vi "CH_LM Globals Debug-Status.vi"() -> ()   [LabVIEW 2017, in "CH_LM App.lvlib"]
uses:
  CH_LM App.lvlib
panel:
  in  "Load Reference":refnum<vi>
  out "Log Counter":i32
  out "GUI Counter":i32
  out "Calculate Counter":i32
  out "Fetch Counter":i32
  out "Callback Counter":i32
  out "Bytes per Element - Trend":i32
  out "Bytes per Element - Log":i32
  out "Bytes per Element - Stream":i32
  in  "My Reference":refnum<vi>
  out "History Array Size":i32
  out "Log Queue # Elements":i32
  out "Trend Queue # Elements":i32
  out "Stream Queue # Elements":i32
  out "Variant Stream Packet Bytes":i32
  # "Coherent LabMax\nStreaming Data Diagnostic Tool"
  # "Asynchronous callback\ndelivers data driven\nby the ActiveX control"
  # "In streaming mode the stream\ncallback converts variant data\nto LabVIEW cluster and\nputs on the stream queue"
  # "LabMax GUI\nVI"
  # "Calculated Trends\nVI"
  # "Log Data\nVI"
  # "Fetch Data\nVI"
  # "Stream Callback\nVI"
  # "Coherent\nActiveX Control"
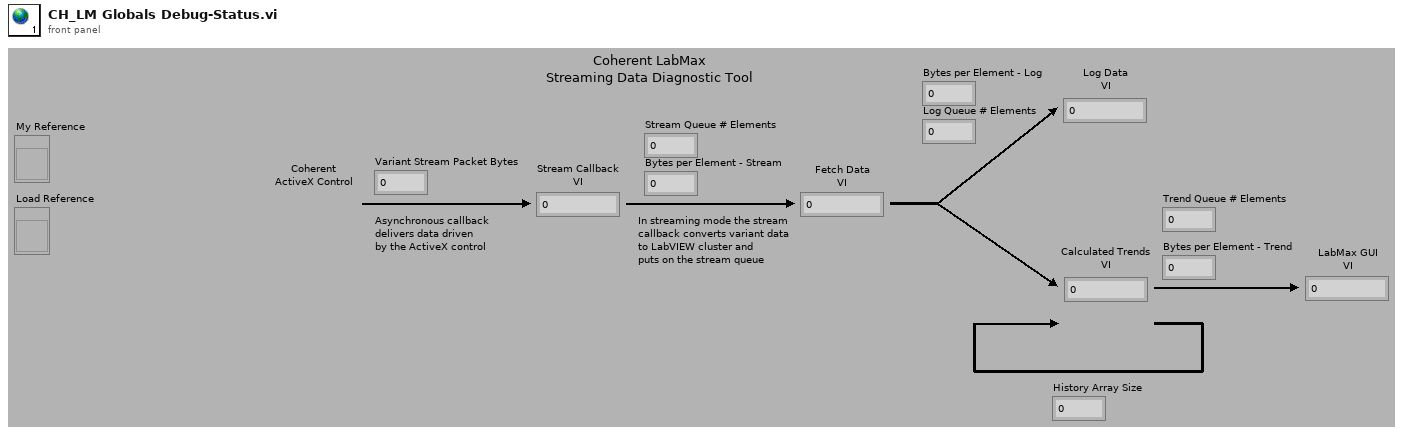
[diagram p1: front panel]
diagram:
